vi "Abort.vi"(11 "MessengerMCPU in":refnum<class "MessengerMCPU.lvclass">) -> (3 "MessengerMCPU out":refnum<class "MessengerMCPU.lvclass">)   [LabVIEW 2019, in "MessengerM.lvlib" / "MessengerMCPU.lvclass"]
uses:
  MessengerMCPU.lvclass
  SubChannelCPU/SubChannelCPU.lvclass
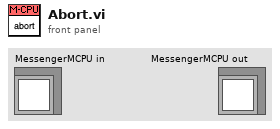
[diagram p1: front panel]
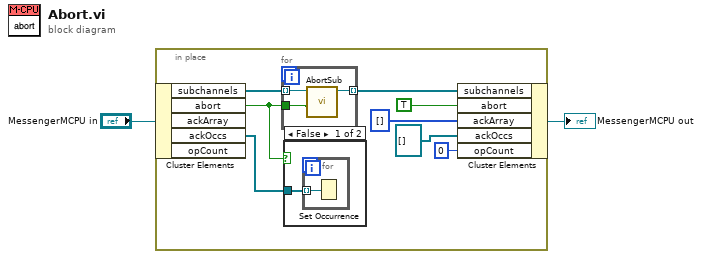
[diagram p0: block diagram]
diagram:
  n1 = in-place {
    n2 = in-place-cluster #1("MessengerMCPU in") -> ("subchannels"=w10:refnum<class "SubChannelCPU.lvclass">[], "abort"=w6:bool, "ackOccs"=w5:refnum<k4>[])  [unwired: 2 out]
    n3 = for {
      tunnel: w10 -> [w15] mode=indexing
      tunnel: [w14] -> w9 mode=indexing
      tunnel: w6 -> [w13]
      n4 = call-dynamic "AbortSub.vi"("aborted"=w13, "SubChannel in"=w15) -> ("SubChannel out"=w14:refnum<class "SubChannelCPU.lvclass">)  [unwired: 9 in]
    }
    n5 = case shown="False" w6 {
      tunnel: w5 -> [w11 _]
      frame False {
        n6 = for {
          tunnel: w11 -> [w12] mode=indexing
          n7 = Set Occurrence(w12) -> ()
        }
      }
      frame True {
      }
    }
    n8 = in-place-cluster #1("subchannels"=w9, "abort"=TRUE, "ackArray"=u32[] [], "ackOccs"=refnum<k4>[] [], "opCount"=u32 0) -> (→"MessengerMCPU out":refnum<class "MessengerMCPU.lvclass">)
  }
